vi "sensor_integration_v3.vi"() -> ()   [LabVIEW 2021]
uses:
  controls/sensirion_flow_sensor_data.ctl
  65c7c016-c5e7-4ca0-8b30-908e1d77d521.vi
  <vilib>/Analysis/baseanly.llb/Mean (DBL).vi
  <vilib>/Instr/_visa.llb/VISA Configure Serial Port (Instr).vi
  <vilib>/Analysis/NI_AALBase.lvlib
panel:
  in  "read byte count (512)":u32=512
  in  "baud rate (576000)":u32=576000
  out "read buffer":string
  out "last loop time, ms":dbl
  out "mean refresh rate, Hz, n=50":dbl
  in  "loop delay, ms (0)":u32
  in  "expected num sensors (12)":i32=12
  out "sensor data array 7 - 12":T1[](array[typedef])=[{"flow rate \n(mL/min)"=0.0, "flow val. status"=FALSE, "temp.\n(C)"=0.0, "temp. val status"=FALSE, "air in \nline?"=FALSE, "high \nflow?"=FALSE, "flag. val status"=FALSE}, {"flow rate \n(mL/min)"=0.0, "flow val. status"=FALSE, "temp.\n(C)"=0.0, "temp. val status"=FALSE, "air in \nline?"=FALSE, "high \nflow?"=FALSE, "flag. val status"=FALSE}, {"flow rate \n(mL/min)"=0.0, "flow val. status"=TRUE, "temp.\n(C)"=0.0, "temp. val status"=TRUE, "air in \nline?"=FALSE, "high \nflow?"=FALSE, "flag. val status"=TRUE}, {"flow rate \n(mL/min)"=0.0, "flow val. status"=TRUE, "temp.\n(C)"=0.0, "temp. val status"=TRUE, "air in \nline?"=FALSE, "high \nflow?"=FALSE, "flag. val status"=TRUE}, {"flow rate \n(mL/min)"=0.0, "flow val. status"=TRUE, "temp.\n(C)"=0.0, "temp. val status"=TRUE, "air in \nline?"=FALSE, "high \nflow?"=FALSE, "flag. val status"=TRUE}, {"flow rate \n(mL/min)"=0.0, "flow val. status"=TRUE, "temp.\n(C)"=0.0, "temp. val status"=TRUE, "air in \nline?"=FALSE, "high \nflow?"=FALSE, "flag. val status"=TRUE}, {"flow rate \n(mL/min)"=0.0, "flow val. status"=TRUE, "temp.\n(C)"=0.0, "temp. val status"=TRUE, "air in \nline?"=FALSE, "high \nflow?"=FALSE, "flag. val status"=TRUE}, {"flow rate \n(mL/min)"=0.0, "flow val. status"=TRUE, "temp.\n(C)"=0.0, "temp. val status"=TRUE, "air in \nline?"=FALSE, "high \nflow?"=FALSE, "flag. val status"=TRUE}, {"flow rate \n(mL/min)"=0.0, "flow val. status"=TRUE, "temp.\n(C)"=0.0, "temp. val status"=TRUE, "air in \nline?"=FALSE, "high \nflow?"=FALSE, "flag. val status"=TRUE}, {"flow rate \n(mL/min)"=0.0, "flow val. status"=TRUE, "temp.\n(C)"=0.0, "temp. val status"=TRUE, "air in \nline?"=FALSE, "high \nflow?"=FALSE, "flag. val status"=TRUE}, {"flow rate \n(mL/min)"=0.0, "flow val. status"=TRUE, "temp.\n(C)"=0.0, "temp. val status"=TRUE, "air in \nline?"=FALSE, "high \nflow?"=FALSE, "flag. val status"=TRUE}, {"flow rate \n(mL/min)"=0.0, "flow val. status"=TRUE, "temp.\n(C)"=0.0, "temp. val status"=TRUE, "air in \nline?"=FALSE, "high \nflow?"=FALSE, "flag. val status"=TRUE}] {"temp.\n(C)" scale=20.0..30.0 scale format="%#_3g"; "flow rate \n(mL/min)" scale=0.0..4.0}
  out "sensor data array 1 - 6":T1[](array[typedef])=[{"flow rate \n(mL/min)"=0.0, "flow val. status"=FALSE, "temp.\n(C)"=0.0, "temp. val status"=FALSE, "air in \nline?"=FALSE, "high \nflow?"=FALSE, "flag. val status"=FALSE}, {"flow rate \n(mL/min)"=0.0, "flow val. status"=FALSE, "temp.\n(C)"=0.0, "temp. val status"=FALSE, "air in \nline?"=FALSE, "high \nflow?"=FALSE, "flag. val status"=FALSE}, {"flow rate \n(mL/min)"=0.0, "flow val. status"=TRUE, "temp.\n(C)"=0.0, "temp. val status"=TRUE, "air in \nline?"=FALSE, "high \nflow?"=FALSE, "flag. val status"=TRUE}, {"flow rate \n(mL/min)"=0.0, "flow val. status"=TRUE, "temp.\n(C)"=0.0, "temp. val status"=TRUE, "air in \nline?"=FALSE, "high \nflow?"=FALSE, "flag. val status"=TRUE}, {"flow rate \n(mL/min)"=0.0, "flow val. status"=TRUE, "temp.\n(C)"=0.0, "temp. val status"=TRUE, "air in \nline?"=FALSE, "high \nflow?"=FALSE, "flag. val status"=TRUE}, {"flow rate \n(mL/min)"=0.0, "flow val. status"=TRUE, "temp.\n(C)"=0.0, "temp. val status"=TRUE, "air in \nline?"=FALSE, "high \nflow?"=FALSE, "flag. val status"=TRUE}, {"flow rate \n(mL/min)"=0.0, "flow val. status"=TRUE, "temp.\n(C)"=0.0, "temp. val status"=TRUE, "air in \nline?"=FALSE, "high \nflow?"=FALSE, "flag. val status"=TRUE}, {"flow rate \n(mL/min)"=0.0, "flow val. status"=TRUE, "temp.\n(C)"=0.0, "temp. val status"=TRUE, "air in \nline?"=FALSE, "high \nflow?"=FALSE, "flag. val status"=TRUE}, {"flow rate \n(mL/min)"=0.0, "flow val. status"=TRUE, "temp.\n(C)"=0.0, "temp. val status"=TRUE, "air in \nline?"=FALSE, "high \nflow?"=FALSE, "flag. val status"=TRUE}, {"flow rate \n(mL/min)"=0.0, "flow val. status"=TRUE, "temp.\n(C)"=0.0, "temp. val status"=TRUE, "air in \nline?"=FALSE, "high \nflow?"=FALSE, "flag. val status"=TRUE}, {"flow rate \n(mL/min)"=0.0, "flow val. status"=TRUE, "temp.\n(C)"=0.0, "temp. val status"=TRUE, "air in \nline?"=FALSE, "high \nflow?"=FALSE, "flag. val status"=TRUE}, {"flow rate \n(mL/min)"=0.0, "flow val. status"=TRUE, "temp.\n(C)"=0.0, "temp. val status"=TRUE, "air in \nline?"=FALSE, "high \nflow?"=FALSE, "flag. val status"=TRUE}] {"temp.\n(C)" scale=20.0..30.0 scale format="%#_3g"; "flow rate \n(mL/min)" scale=0.0..3.0}
  out "error out":errorcluster
  out "return byte count":u32
  in  "stop program":bool
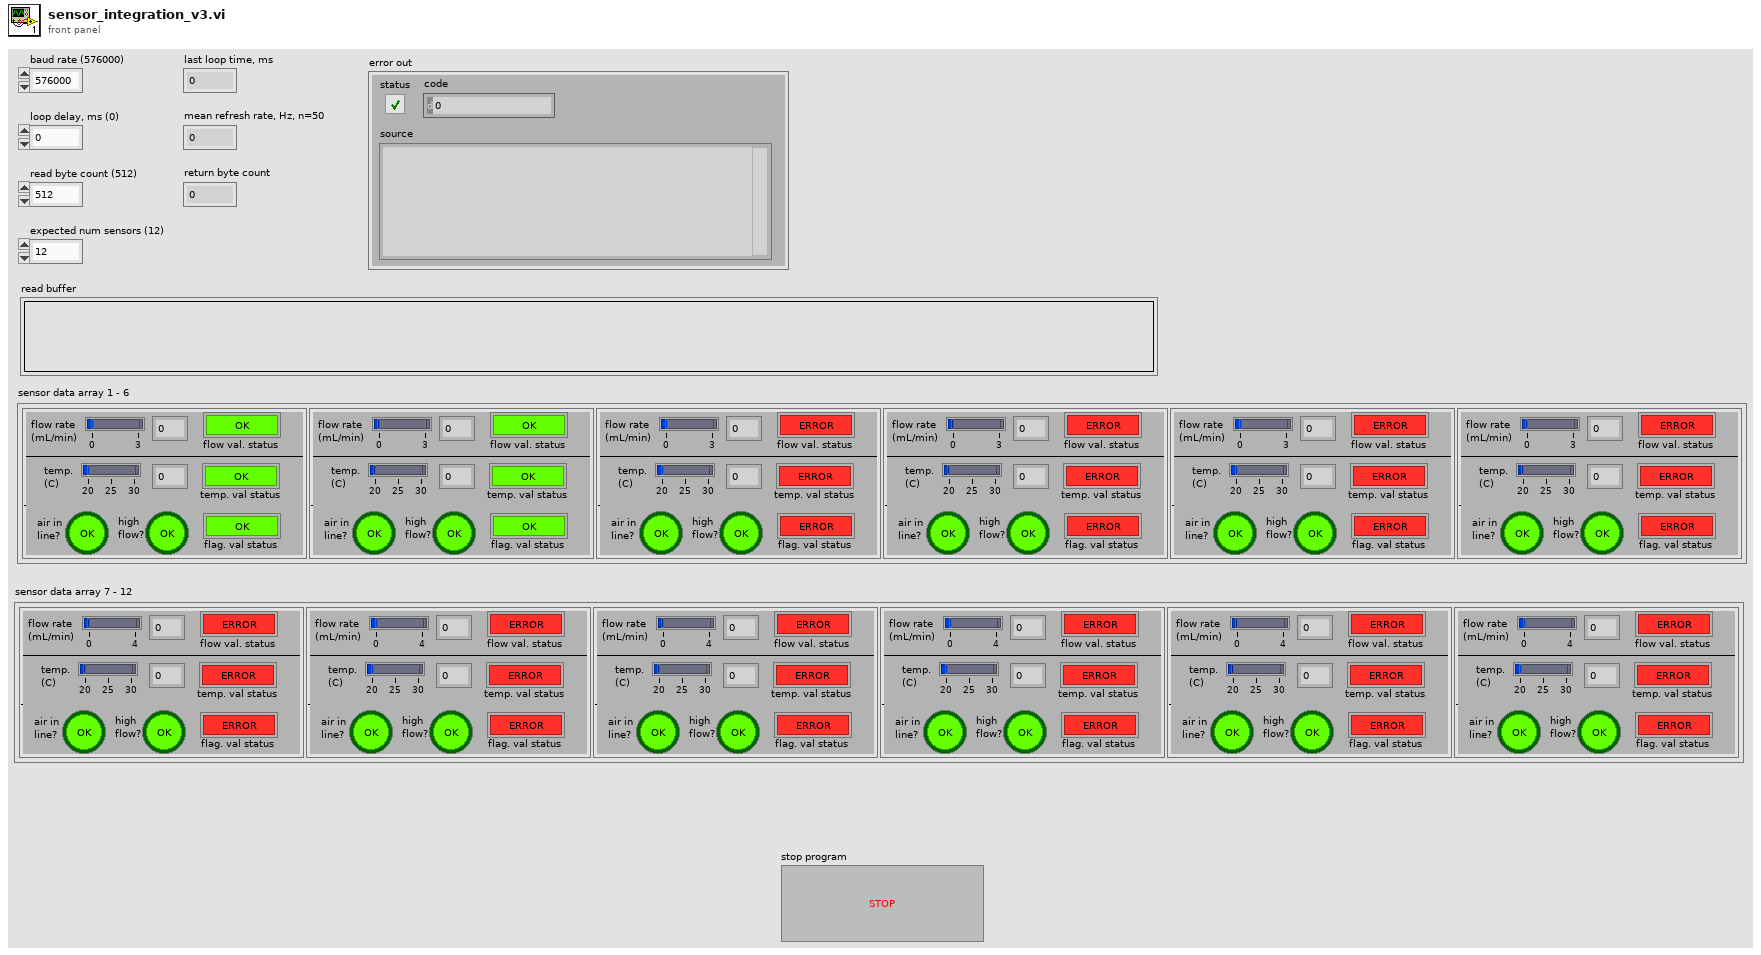
[diagram p1: front panel]
types:
  T1 = typedef "sensirion_flow_sensor_data.ctl" = cluster{"flow rate \n(mL/min)":dbl, "flow val. status":bool, "temp.\n(C)":dbl, "temp. val status":bool, "air in \nline?":bool, "high \nflow?":bool, "flag. val status":bool}
  T2 = enum8{"Enabled", "Disabled", "Disabled and Grayed Out"}
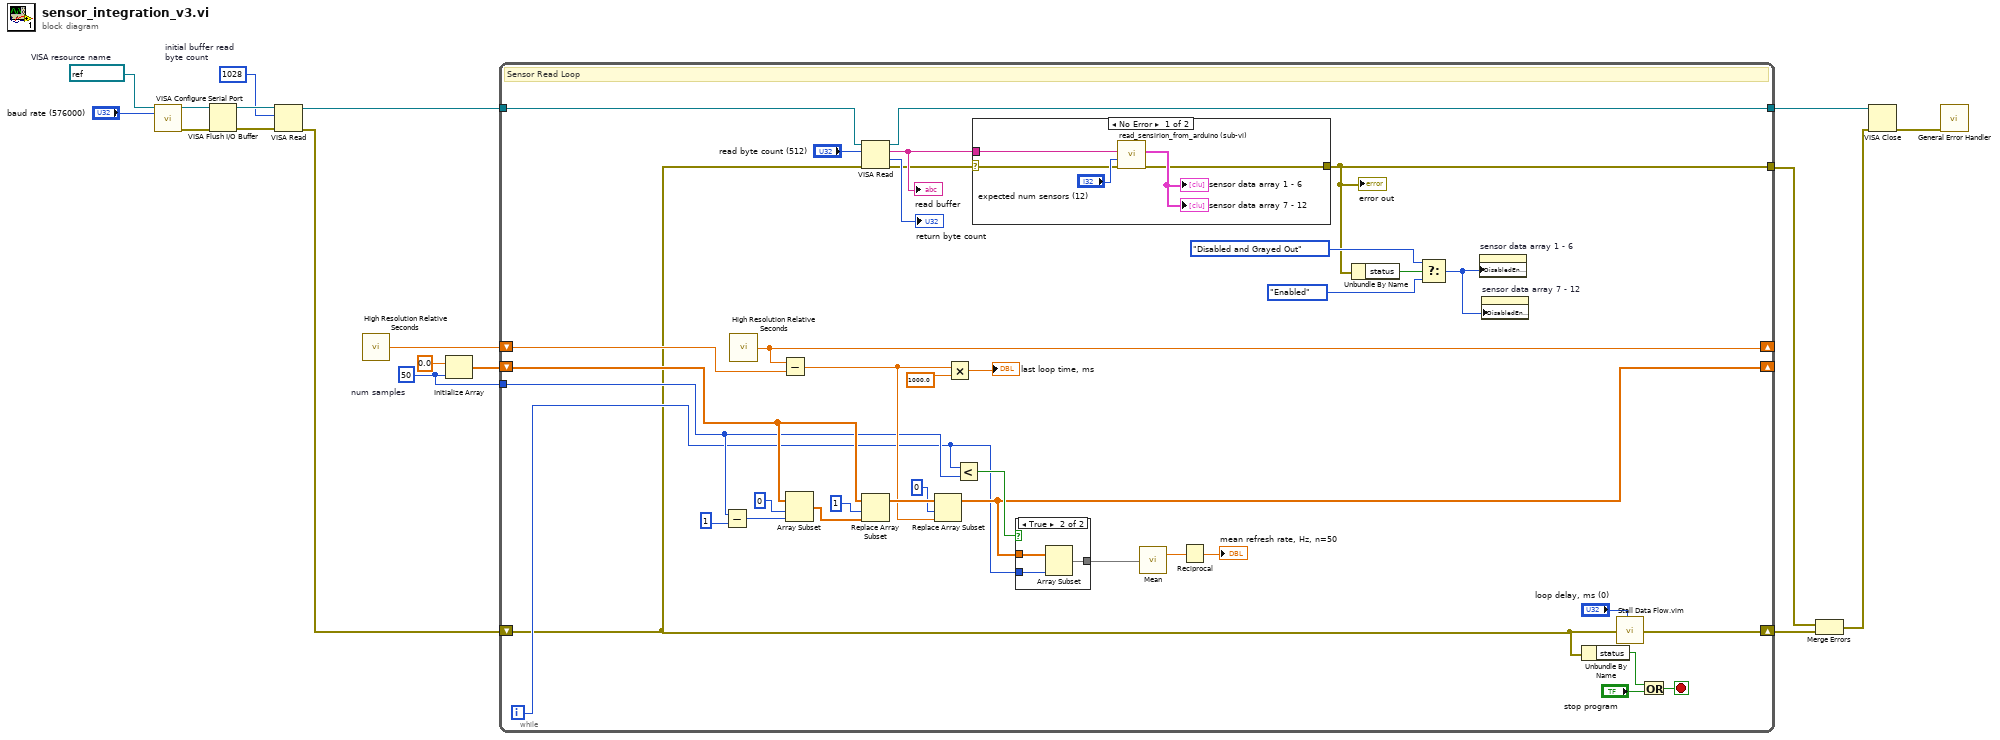
[diagram p0: block diagram]
diagram:
  w6 = 50  # num samples
  w10 = u32 1028  # initial buffer read byte count
  w16 = refnum<visa-resource-name> "COM3"  # VISA resource name
  n1 = call-poly "VISA Configure Serial Port"("VISA resource name"=w16, "baud rate (9600)"="baud rate (576000)") -> ("VISA resource name out"=w14:refnum<visa-resource-name>, "error out"=w13:errorcluster)  [unwired: 12 in]
  n2 = VISA Flush I/O Buffer(VISA resource name=w14, error in (no error)=w13) -> (VISA resource name out=w11:refnum<visa-resource-name>, error out=w12:errorcluster)  [unwired: 1 in]
  n3 = VISA Read(VISA resource name=w11, byte count=w10, error in (no error)=w12) -> (VISA resource name out=w15:refnum<visa-resource-name>, error out=w7:errorcluster)  [unwired: 2 out]
  n4 = call <vilib>:"High Resolution Relative Seconds.vi"() -> ("relative seconds"=w5:dbl)
  n5 = Initialize Array(0.0 ("element"), w6) -> (w8:dbl[])
  n6 = while {
    tunnel: w15 -> [w43]
    tunnel: [w39] -> w18
    shift-right: [w54] -> _
    shift-left: w5 -> [w53]
    shift-right: [w35] -> _
    shift-left: w8 -> [w49]
    shift-right: [w20] -> w3
    shift-left: w7 -> [w24]
    tunnel: w6 -> [w37]
    tunnel: [w28] -> w2
    i -> [w34]
    stop <- w27 stop-if-true
    # "Sensor Read Loop"
    n7 = Subtract(x=w37, y=1) -> (x-y=w47:i32)
    n8 = call <vilib>:"High Resolution Relative Seconds.vi"() -> ("relative seconds"=w54:dbl)
    n9 = Subtract(x=w54, y=w53) -> (x-y=w45:dbl)
    n10 = Array Subset(array=w49, index=0, length=w47) -> (w52:dbl[])
    n11 = VISA Read(VISA resource name=w43, byte count="read byte count (512)", error in (no error)=w24) -> (VISA resource name out=w39:refnum<visa-resource-name>, read buffer=w42:string, return count=→"return byte count":u32, error out=w38:errorcluster)
    "read buffer" <- w42
    n12 = Replace Array Subset(array=w49, new element=w52, index=1) -> (w46:dbl[])
    n13 = Replace Array Subset(array=w46, new element=w45, index=0) -> (w35:dbl[])
    n14 = Multiply(x=w45, y=1000.0) -> (x*y=→"last loop time, ms":dbl)
    n15 = Less?(x=w34, y=w37) -> (x < y?=w36:bool)
    n16 = case shown="No Error" w38 {
      selector: w38 -> [w60 w65]
      tunnel: [w62 w65] -> w28
      tunnel: w42 -> [w61 _]
      frame No Error {
        n17 = call "read_sensirion_from_arduino (sub-vi).vi"("error in"=w60, "expected num sensors (12)"="expected num sensors (12)", "serial buffer in"=w61) -> ("error out"=w62:errorcluster, "sensor data array"=→"sensor data array 1 - 6" →"sensor data array 7 - 12":T1[])  [unwired: 7 in]
      }
      frame Error {
      }
    }
    "error out" <- w28
    n18 = case shown="True" w36 {
      tunnel: w35 -> [w56 w59]
      tunnel: w34 -> [_ w58]
      tunnel: [w56 w57] -> w33
      frame False {
      }
      frame True {
        n19 = Array Subset(array=w59, length=w58) -> (w57:dbl[])  [unwired: 1 in]
      }
    }
    n20 = call-poly <vilib>:"Mean.vi"("X"=w33) -> ("mean"=w32:dbl)  [unwired: 1 out]
    n21 = Reciprocal(x=w32) -> (1/x=→"mean refresh rate, Hz, n=50":dbl)
    n22 = Unbundle By Name(w28) -> ("status"=w31:bool)
    n23 = Select(t=T2."Disabled and Grayed Out" ("Disabled"), s=w31, f=T2."Enabled" ("Disabled")) -> (s? t:f=w29:T2)
    n24 = property on="sensor data array 1 - 6" class="Arr (strict)"("DisabledEnum"=w29) -> ()  [unwired: 2 in, 2 out]
    n25 = property on="sensor data array 7 - 12" class="Arr (strict)"("DisabledEnum"=w29) -> ()  [unwired: 2 in, 2 out]
    n26 = Unbundle By Name(w24) -> ("status"=w25:bool)
    n27 = call "Stall Data Flow.vim"("value in"=w24, "milliseconds to wait"="loop delay, ms (0)") -> ("value out"=w20:errorcluster)  [unwired: 1 out]
    n28 = Or(x=w25, y="stop program") -> (x .or. y?=w27:bool)
  }
  n29 = Merge Errors(w2, w3) -> (w1:errorcluster)
  n30 = VISA Close(VISA resource name=w18, error in (no error)=w1) -> (error out=w4:errorcluster)
  n31 = call <vilib>:"General Error Handler.vi"("error in (no error)"=w4) -> ()  [unwired: 10 in, 5 out]
